vi "Get Daemon Termination Status.vi"(8 "error in (no error)":errorcluster, 11 "WAMP Client in":refnum<class "WAMP Client.lvclass">) -> (0 "error out":errorcluster, 1 "Termination Reason":T1={"Reason"=enum."Goodbye Received", "Reason URI"="wamp.error.protocol_violation", "Message"=""}, 2 "Terminate?":bool, 3 "WAMP Client out":refnum<class "WAMP Client.lvclass">)   [LabVIEW 2020, in "wamplv.lvlib" / "WAMP Client.lvclass"]
uses:
  WAMP Client.lvclass
  API/TypeDefs/Termination Reason.ctl
  TypeDef/Termination Reason Enum.ctl
  WAMP Client.lvclass/WAMP Client.ctl
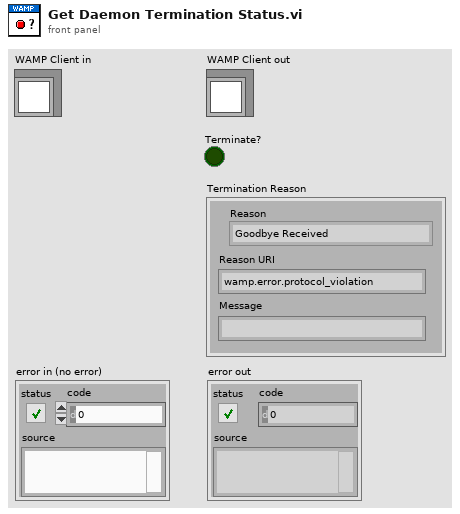
[diagram p1: front panel]
types:
  T1 = typedef "wamplv.lvlib/WAMP Client.lvclass/Termination Reason.ctl" = cluster{"Reason":T2, "Reason URI":string, "Message":string}
  T2 = typedef "wamplv.lvlib/WAMP Client.lvclass/Termination Reason Enum.ctl" = enum16{"Goodbye Received", "Abort Received", "Send Goodbye", "Send Abort", "Read Loop Failure", "Write Loop Failure", "Message Loop Failure"}
  T3 = typedef "wamplv.lvlib/WAMP Client.lvclass/Termination Request.ctl" = cluster{"Terminate?":bool, "Termination Reason":T1}
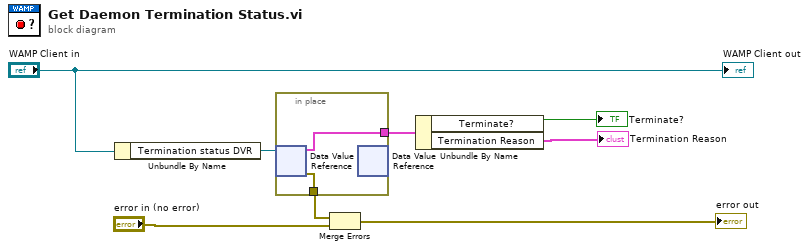
[diagram p0: block diagram]
diagram:
  n1 = Unbundle By Name("WAMP Client in") -> ("Termination status DVR"=w4:refnum<data-value>)
  n2 = in-place "In Place Element Structure" {
    in-place-border: [w10] -> w2
    in-place-border: [w9] -> w1
    n3 = in-place-dvr #1(w4) -> (w10:T3, w9:errorcluster)
    n4 = in-place-dvr #1() -> ()  [unwired: 1 in, 2 out]
  }
  n5 = Merge Errors(w1, "error in (no error)") -> (→"error out":errorcluster)
  n6 = Unbundle By Name(w2) -> ("Terminate?"=→"Terminate?":bool, "Termination Reason"=→"Termination Reason":T1)
  "WAMP Client out" <- "WAMP Client in"
